vi "read_db_for_dcs_spot.vi"(8 "error in (no error)":errorcluster, 11 "Constraints":T2) -> (0 "error out":errorcluster, 3 "DCS Spot Array":T1[](array[typedef]))   [LabVIEW 2013]
uses:
  Controls/DCSConstraints.ctl
  Controls/dcs_spot.ctl
  <vilib>/addons/database/_DB Variant To Data/Database Variant To Data.xnode
panel:
  out "SQL Query Syntax":string
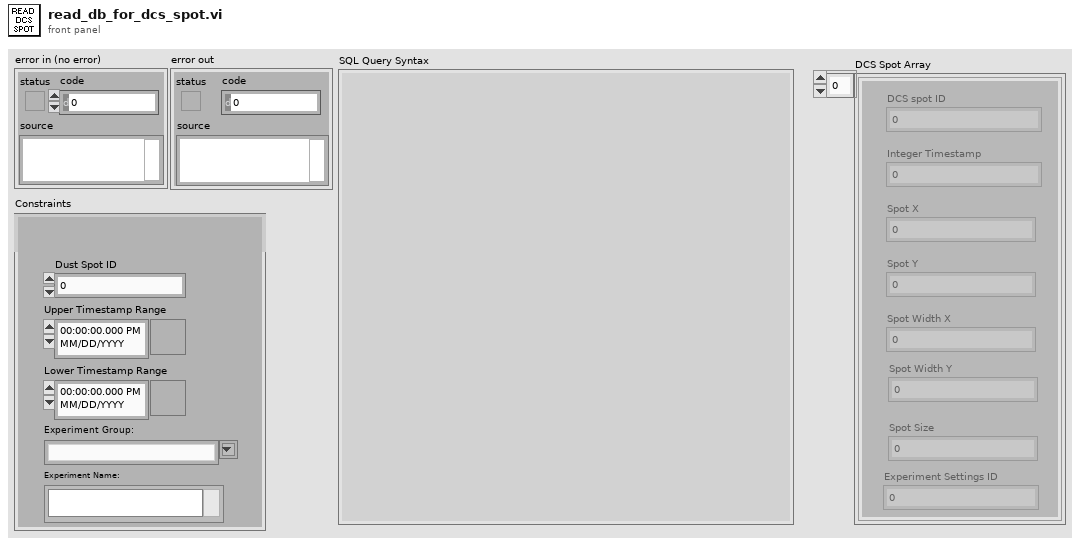
[diagram p1: front panel]
types:
  T1 = typedef "dcs_spot.ctl" = cluster{"DCS spot ID":i32, "Integer Timestamp":i64, "Spot X":dbl, "Spot Y":dbl, "Spot Width X":dbl, "Spot Width Y":dbl, "Spot Size":i32, "Experiment Settings ID":i32}
  T2 = typedef "DCSConstraints.ctl" = cluster{"Upper Timestamp Range":timestamp, "Lower Timestamp Range":timestamp, "Experiment Group:":string, "Experiment Name:":i32[], "name array":string[], "Dust Spot ID":dbl}
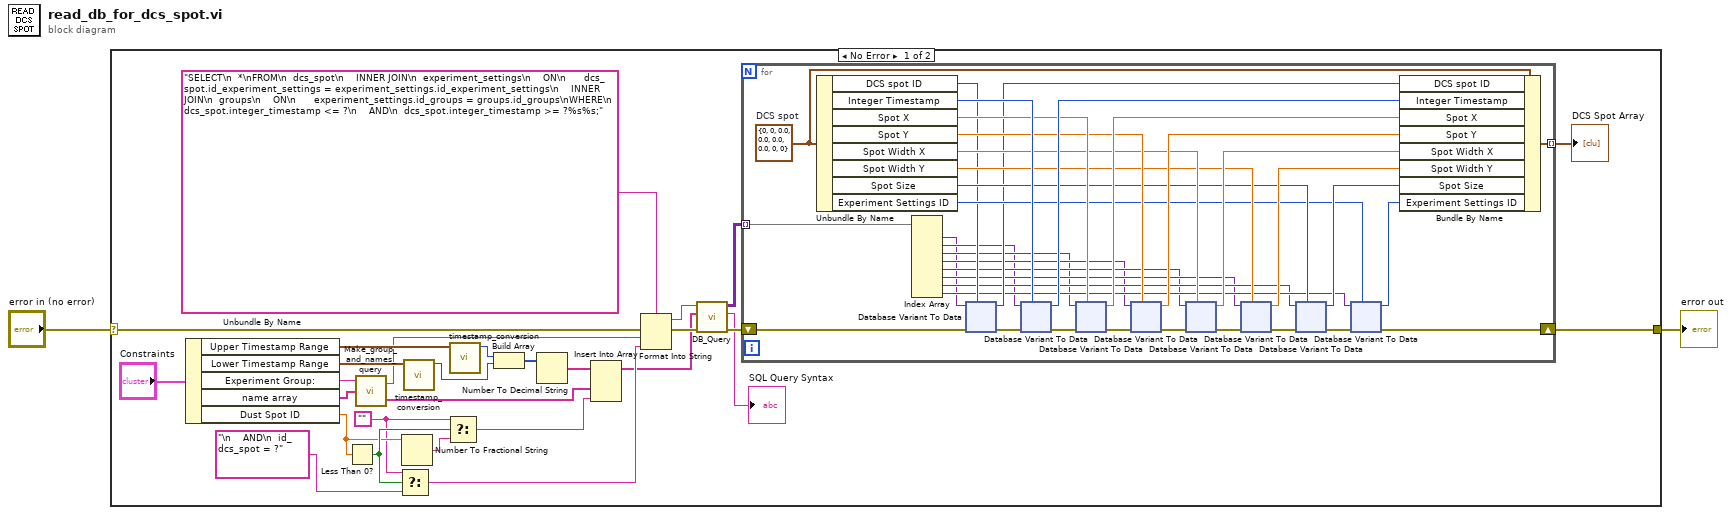
[diagram p0: block diagram]
diagram:
  n1 = case shown="No Error" "error in (no error)" {
    selector: "error in (no error)" -> [w5 w323]
    tunnel: [w4 w323] -> w1
    frame No Error {
      w3 = ""
      n2 = Unbundle By Name("Constraints") -> ("Upper Timestamp Range"=w29:timestamp, "Lower Timestamp Range"=w30:timestamp, "Experiment Group:"=w22:string, "name array"=w21:string[], "Dust Spot ID"=w15:dbl)
      n3 = Less Than 0?(x=w15) -> (x < 0?=w16:bool)
      n4 = call "Make_group_and_names_query.vi"("Name Array"=w21, "Group  Name"=w22) -> ("Parameters"=w20:string[], "Group and Names Query"=w17:string)  [unwired: 1 in]
      n5 = Select(t=w3, s=w16, f="\n    AND\n  id_dcs_spot = ?" ("string")) -> (s? t:f=w12:string)
      n6 = Number To Fractional String(number=w15) -> (F-format string=w14:string)  [unwired: 3 in]
      n7 = call "timestamp_conversion.vi"("Time Stamp"=w30) -> ("Integer Time"=w24:i64)  [unwired: 8 in, 1 out]
      n8 = Select(t=w3, s=w16, f=w14) -> (s? t:f=w13:string)
      n9 = call "timestamp_conversion.vi"("Time Stamp"=w29) -> ("Integer Time"=w25:i64)  [unwired: 8 in, 1 out]
      n10 = Build Array(w25, w24) -> (w26:i64[])
      n11 = Number To Decimal String(number=w26) -> (decimal integer string=w23:string[])  [unwired: 1 in]
      n12 = Insert Into Array(array=w23, new element #1=w20, new element #2=w13) -> (w6:string[])  [unwired: 1 in]
      n13 = Format Into String(format string="SELECT\n  *\nFROM\n  dcs_spot\n    INNER JOIN\n  experiment_settings\n    ON\n      dcs_spot.id_experiment_settings = experiment_settings.id_experiment_settings\n    INNER JOIN\n  groups\n    ON\n      experiment_settings.id_groups = groups.id_groups\nWHERE\n  dcs_spot.integer_timestamp <= ?\n    AND\n  dcs_spot.integer_timestamp >= ?%s%s;", error in=w5, w17, w12) -> (resulting string=w7:string, error out=w10:errorcluster)  [unwired: 1 in]
      n14 = call "DB_Query.vi"("error in (no error)"=w10, "Parameters"=w6, "Parameterized Query"=w7) -> ("error out"=w11:errorcluster, "Query in Standard Format"=→"SQL Query Syntax":string, "Results"=w8:variant[][])  [unwired: 6 in]
      n15 = for {
        shift-right: [w42] -> w4
        shift-left: w11 -> [w66]
        tunnel: [w62] -> w27 mode=indexing
        tunnel: w8 -> [w31] mode=indexing
        w60 = T1 {"DCS spot ID"=0, "Integer Timestamp"=0, "Spot X"=0.0, "Spot Y"=0.0, "Spot Width X"=0.0, "Spot Width Y"=0.0, "Spot Size"=0, "Experiment Settings ID"=0}  # DCS spot
        n16 = Unbundle By Name(w60) -> ("DCS spot ID"=w41:i32, "Integer Timestamp"=w59:i64, "Spot X"=w57:dbl, "Spot Y"=w55:dbl, "Spot Width X"=w53:dbl, "Spot Width Y"=w50:dbl, "Spot Size"=w48:i32, "Experiment Settings ID"=w46:i32)
        n17 = Index Array(array=w31) -> (element #1=w32:variant, element #2=w33:variant, element #3=w34:variant, element #4=w35:variant, element #5=w36:variant, element #6=w37:variant, element #7=w38:variant, element #8=w39:variant)  [unwired: 8 in]
        n18 = xnode "Database Variant To Data"("database variant"=w32, "error in (no error)"=w66, "type"=w41) -> ("data"=w40:i32, "error out"=w65:errorcluster)
        n19 = xnode "Database Variant To Data"("database variant"=w33, "error in (no error)"=w65, "type"=w59) -> ("data"=w58:i64, "error out"=w64:errorcluster)
        n20 = xnode "Database Variant To Data"("database variant"=w34, "error in (no error)"=w64, "type"=w57) -> ("data"=w56:dbl, "error out"=w63:errorcluster)
        n21 = xnode "Database Variant To Data"("database variant"=w35, "error in (no error)"=w63, "type"=w55) -> ("data"=w54:dbl, "error out"=w61:errorcluster)
        n22 = xnode "Database Variant To Data"("database variant"=w36, "error in (no error)"=w61, "type"=w53) -> ("data"=w52:dbl, "error out"=w51:errorcluster)
        n23 = xnode "Database Variant To Data"("database variant"=w37, "error in (no error)"=w51, "type"=w50) -> ("data"=w49:dbl, "error out"=w44:errorcluster)
        n24 = xnode "Database Variant To Data"("database variant"=w38, "error in (no error)"=w44, "type"=w48) -> ("data"=w47:i32, "error out"=w43:errorcluster)
        n25 = xnode "Database Variant To Data"("database variant"=w39, "error in (no error)"=w43, "type"=w46) -> ("data"=w45:i32, "error out"=w42:errorcluster)
        n26 = Bundle By Name(cluster=w60, "DCS spot ID"=w40, "Integer Timestamp"=w58, "Spot X"=w56, "Spot Y"=w54, "Spot Width X"=w52, "Spot Width Y"=w49, "Spot Size"=w47, "Experiment Settings ID"=w45) -> (w62:T1)
      }
      "DCS Spot Array" <- w27
    }
    frame Error {
    }
  }
  "error out" <- w1
